vi "Get Preferences Archive Path.vi"() -> (0 "path":path)   [LabVIEW 2013]
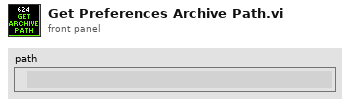
[diagram p1: front panel]
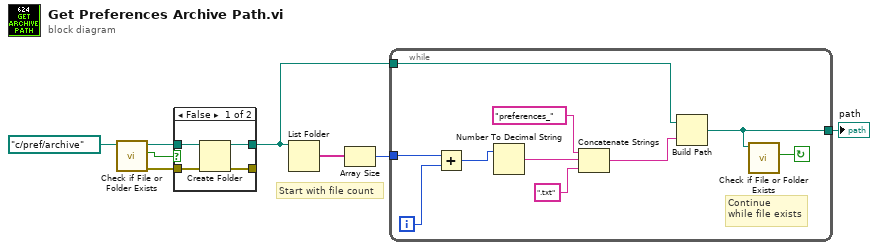
[diagram p0: block diagram]
diagram:
  # "Start with file count"
  n1 = call <vilib>:"Check if File or Folder Exists.vi"("path"=path "c:/pref/archive") -> ("error out"=w4:errorcluster, "file or folder exists?"=w5:bool, "dup path"=w3:path)  [unwired: 8 in]
  n2 = case shown="False" w5 {
    tunnel: w3 -> [w12 w13]
    tunnel: w4 -> [w11 w14]
    tunnel: [w10 w13] -> w1
    tunnel: [w9 w14] -> _
    frame False {
      n3 = Create Folder(path (use dialog)=w12, error in=w11) -> (created path=w10:path, error out=w9:errorcluster)  [unwired: 1 in, 1 out]
    }
    frame True {
    }
  }
  n4 = List Folder(path=w1) -> (filenames=w7:string[])  [unwired: 3 in, 3 out]
  n5 = Array Size(array=w7) -> (size(s)=w6:i32)
  n6 = while {
    tunnel: [w17] -> w8
    tunnel: w6 -> [w22]
    tunnel: w1 -> [w15]
    i -> [w21]
    stop <- w18 continue-if-true
    # "Continue\nwhile file exists"
    n7 = Add(x=w22, y=w21) -> (x+y=w20:i32)
    n8 = Number To Decimal String(number=w20) -> (decimal integer string=w19:string)  [unwired: 1 in]
    n9 = Concatenate Strings("preferences_" ("string"), w19, ".txt" ("string")) -> (w16:string)
    n10 = Build Path(base path=w15, name or relative path=w16) -> (appended path=w17:path)
    n11 = call <vilib>:"Check if File or Folder Exists.vi"("path"=w17) -> ("file or folder exists?"=w18:bool)  [unwired: 8 in, 2 out]
  }
  "path" <- w8
